vi "FTW-STR-Array-Concatenate.vi"(5 "Array of Strings":string[](array[string]), 7 "Format String":string="[%s]") -> (6 "Concatenated String":string)   [LabVIEW 2015]
panel:
  # "Inputs"
  # "Outputs"
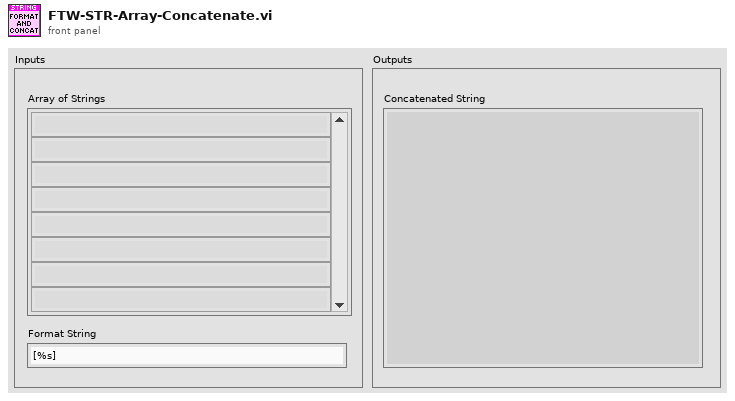
[diagram p1: front panel]
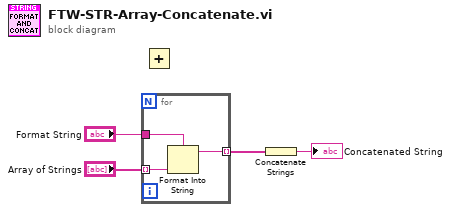
[diagram p0: block diagram]
diagram:
  n1 = for {
    tunnel: "Format String" -> [w6]
    tunnel: "Array of Strings" -> [w7] mode=indexing
    tunnel: [w5] -> w1 mode=indexing
    n2 = Format Into String(format string=w6, w7) -> (resulting string=w5:string)  [unwired: 2 in, 1 out]
  }
  n3 = Add() -> ()  [unwired: 2 in, 1 out]
  n4 = Concatenate Strings(w1) -> (→"Concatenated String":string)
